vi "Teleop.vi"(10 "Match Info":T2={"Autonomous Elapsed Seconds"=0.0, "TeleOp Elapsed Seconds"=0.0, "Disabled Elapsed Seconds"=0.0, "Visited Autonomous"=FALSE, "Visited TeleOp"=FALSE, "Visited Disabled"=FALSE, "Autonomous Settings"={"Autonomous Style"=enum."Independent", "VI Refnum"=refnum}}, 11 "Call Context":T3) -> ()   [LabVIEW 2011]
doc: "This VI is called for each TeleOp packet received from the DS where the robot is not disabled. It is often used to read from the joysticks and update I/O or to update setpoints for timed control loops. It should complete and return within 20 milliseconds or it may miss DS packets."
uses:
  <vilib>/Rock Robotics/WPI/DriverStation/WPI_DriverStationDerivedRobotMode.ctl
  <vilib>/Rock Robotics/WPI/DriverStation/WPI_DriverStationMatch Info.ctl
  <vilib>/Rock Robotics/WPI/Joystick/WPI_JoystickButtonState.ctl
  Robot Global Data.vi
panel:
  in  "rpm fender diff":dbl=900.0
  out "Buttons 2":T1
  in  "dedband":dbl=0.1 step=0.01
  out "drive 2":bool
  out "drive 1":bool
  out "x-y":u32
  in  "Numeric":dbl=0.3
  out "Buttons":T1
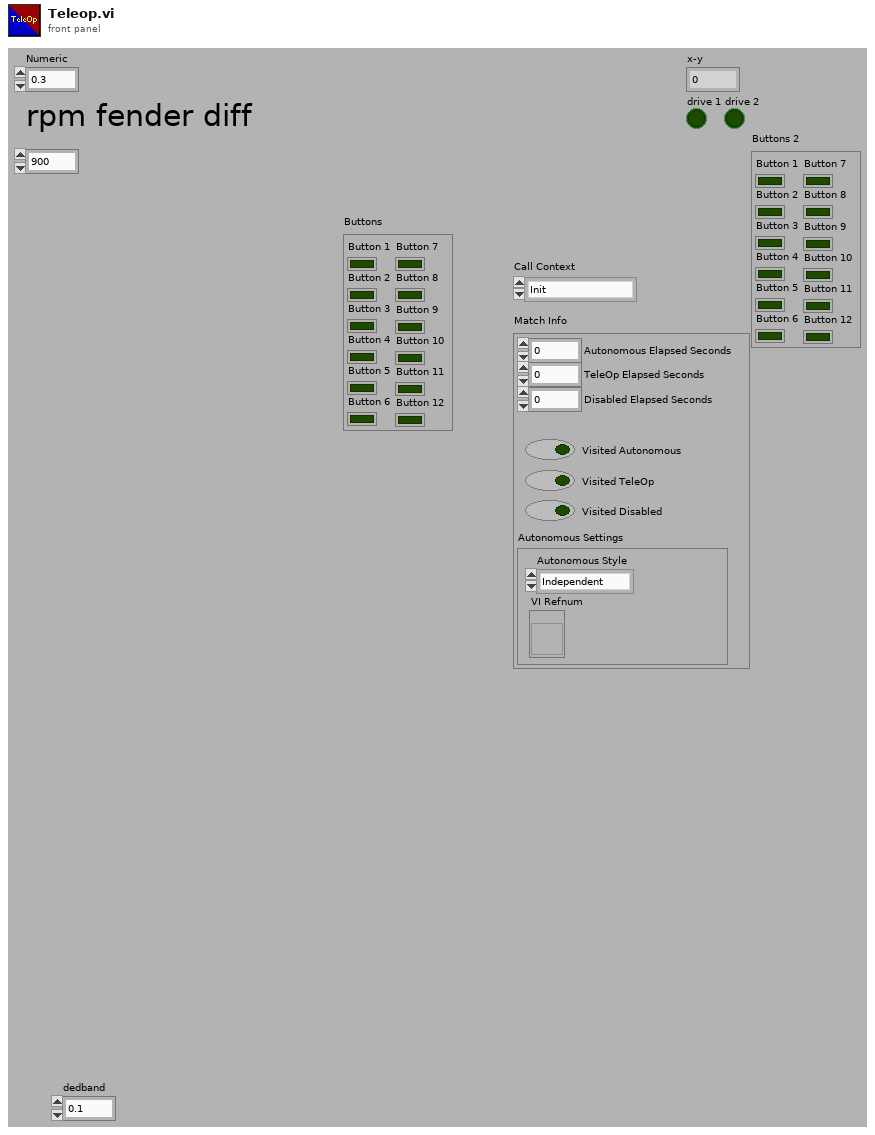
[diagram p1: front panel]
types:
  T1 = typedef "WPI_JoystickButtonState.ctl" = cluster{"Button 1":bool, "Button 2":bool, "Button 3":bool, "Button 4":bool, "Button 5":bool, "Button 6":bool, "Button 7":bool, "Button 8":bool, "Button 9":bool, "Button 10":bool, "Button 11":bool, "Button 12":bool}
  T2 = typedef "WPI_DriverStationMatch Info.ctl" = cluster{"Autonomous Elapsed Seconds":dbl, "TeleOp Elapsed Seconds":dbl, "Disabled Elapsed Seconds":dbl, "Visited Autonomous":bool, "Visited TeleOp":bool, "Visited Disabled":bool, "Autonomous Settings":cluster{"Autonomous Style":enum16{"Iterative", "Independent"}, "VI Refnum":refnum<vi>}}
  T3 = typedef "WPI_DriverStationDerivedRobotMode.ctl" = enum16{"Init", "Execute", "Stop"}
  T4 = typedef "WPI_JoystickDevRef.ctl" = cluster{"Device":T5}
  T5 = typedef "WPI_JoystickDeviceEnum.ctl" = enum16{"USB 1", "USB 2", "USB 3", "USB 4", "Kinect 1", "Kinect 2"}
  T6 = cluster{"axis 1 (x)":dbl, "axis 2 (y)":dbl, "axis 3 (throttle)":dbl, "axis 4":dbl, "axis 5":dbl, "axis 6":dbl}
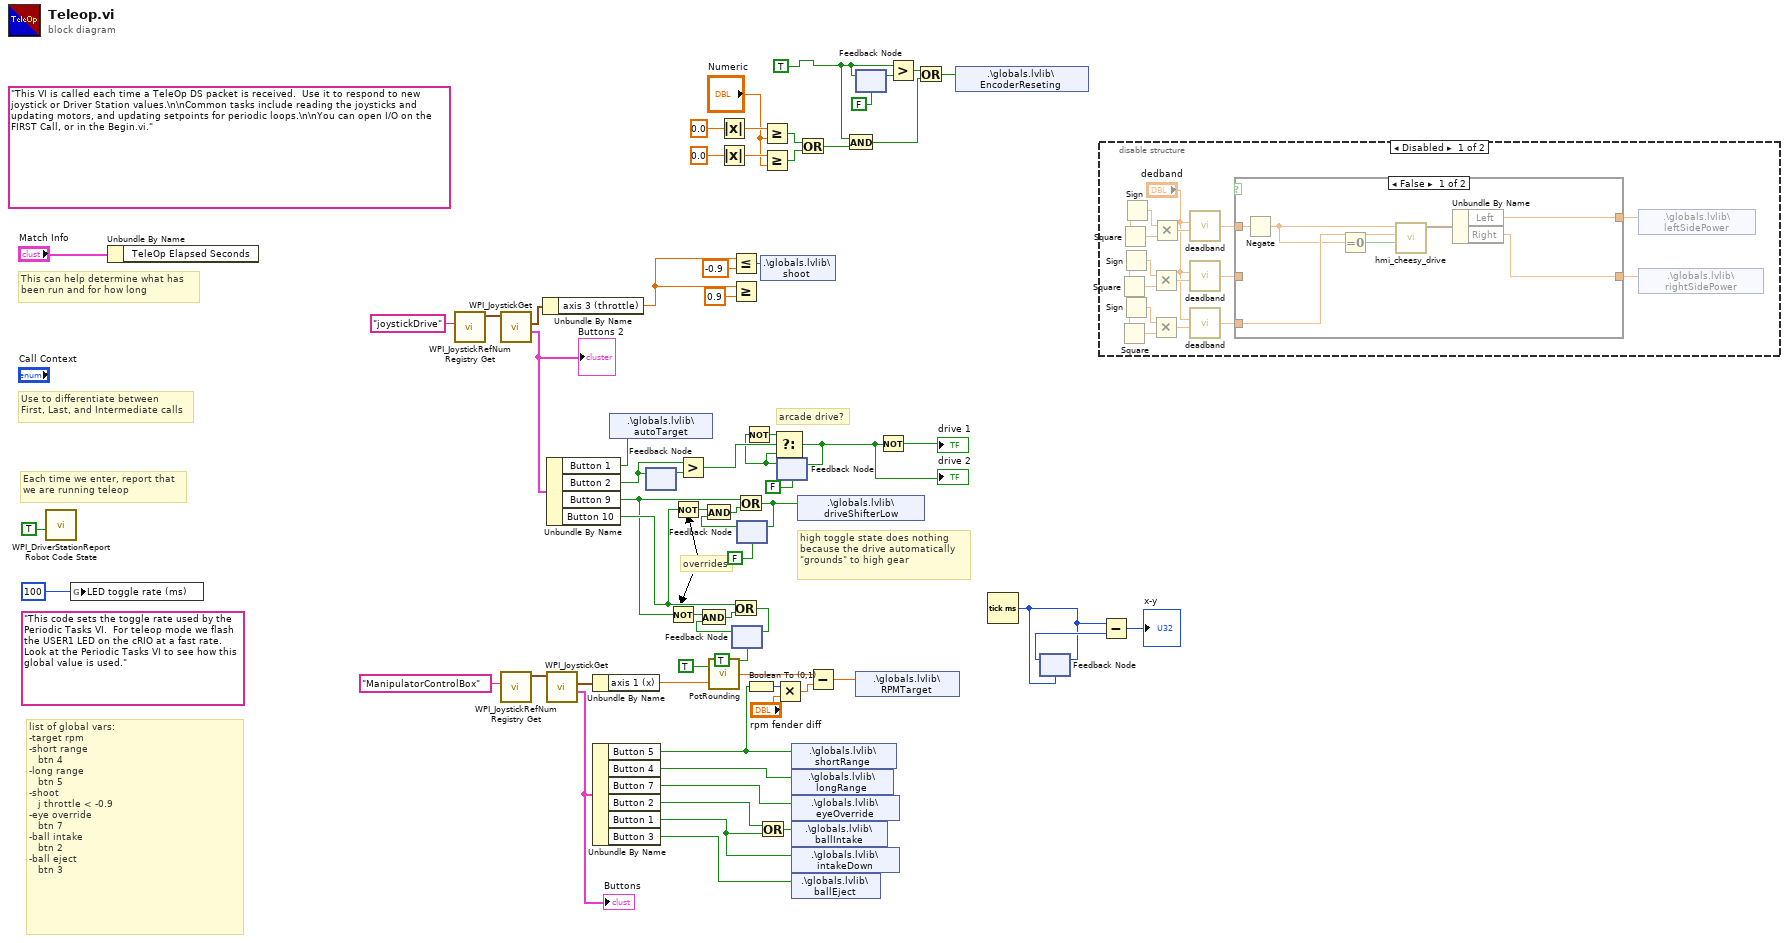
[diagram p0: block diagram]
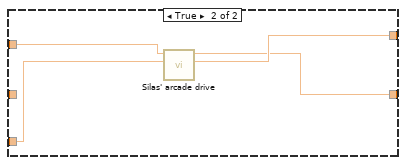
[diagram p2: hidden frame]
diagram:
  w20 = TRUE ("x")
  (unwired) "This code sets the toggle rate used by the Periodic Tasks VI.  For teleop mode we flash the USER1 LED on the cRIO at a fast rate.  Look at the Periodic Tasks VI to see how this global value is used."
  (unwired) "This VI is called each time a TeleOp DS packet is received.  Use it to respond to new joystick or Driver Station values.\n\nCommon tasks include reading the joysticks and updating motors, and updating setpoints for periodic loops.\n\nYou can open I/O on the FIRST Call, or in the Begin.vi."
  # "arcade drive?"
  # "high toggle state does nothing because the drive automatically \"grounds\" to high gear"
  # "overrides"
  # "list of global vars:\n-target rpm\n-short range\n   btn 4\n-long range\n   btn 5\n-shoot\n   j throttle < -0.9\n-eye override\n   btn 7\n-ball intake\n   btn 2\n-ball eject\n   btn 3"
  # "Each time we enter, report that\nwe are running teleop"
  # "Use to differentiate between\nFirst, Last, and Intermediate calls"
  # "This can help determine what has\nbeen run and for how long"
  n1 = call <vilib>:"WPI_DriverStationReport Robot Code State.vi"("TeleOp"=TRUE ("Autonomous")) -> ()  [unwired: 10 in, 1 out]
  n2 = global write "Robot Global Data.vi" "LED toggle rate (ms)"(u32 100 ("LED ms toggle rate")) -> ()
  n3 = Unbundle By Name("Match Info") -> ()  [unwired: 1 out]
  n4 = call <vilib>:"WPI_JoystickRefNum Registry Get.vi"("refnum name"="joystickDrive") -> ("JoystickDevRef"=w62:T4)  [unwired: 9 in, 1 out]
  n5 = call <vilib>:"WPI_JoystickGet.vi"("JoystickDevRef"=w62) -> ("Buttons"=w49:T1, "Axes"=w60:T6)  [unwired: 4 in, 1 out]
  "Buttons 2" <- w49
  n6 = call <vilib>:"WPI_JoystickRefNum Registry Get.vi"("refnum name"="ManipulatorControlBox") -> ("JoystickDevRef"=w61:T4)  [unwired: 9 in, 1 out]
  n7 = Unbundle By Name(w60) -> ("axis 3 (throttle)"=w17:dbl)
  n8 = Unbundle By Name(w49) -> ("Button 1"=w28:bool, "Button 2"=w26:bool, "Button 9"=w25:bool, "Button 10"=w52:bool)
  n9 = call <vilib>:"WPI_JoystickGet.vi"("JoystickDevRef"=w61) -> ("Buttons"=w58:T1, "Axes"=w59:T6)  [unwired: 4 in, 1 out]
  "Buttons" <- w58
  n10 = Unbundle By Name(w59) -> ("axis 1 (x)"=w46:dbl)
  n11 = Unbundle By Name(w58) -> ("Button 5"=w6:bool, "Button 4"=w57:bool, "Button 7"=w7:bool, "Button 2"=w14:bool, "Button 1"=w13:bool, "Button 3"=w12:bool)
  n12 = shared-variable ".\\globals.lvlib\\autoTarget"(w28) -> ()  [unwired: 1 in, 1 out]
  n13 = feedback-in #1(w26) -> ()
  n14 = feedback #1() -> (w27:bool)  [unwired: 1 in]
  n15 = Not(x=w25) -> (.not. x?=w55:bool)
  n16 = Not(x=w52) -> (.not. x?=w54:bool)
  n17 = Greater?(x=w26, y=w27) -> (0:w24:bool)
  n18 = call "PotRounding.vi"("Potentiometer"=w46, "Invert?"=TRUE) -> ("shooter output"=w2:dbl)
  n19 = Absolute Value(x=0.0) -> (abs(x)=w40:dbl)
  n20 = Absolute Value(x=0.0) -> (abs(x)=w39:dbl)
  n21 = Less Or Equal?(x=w17, y=-0.9) -> (x <= y?=w19:bool)
  n22 = Greater Or Equal?(x=w17, y=0.9) -> ()  [unwired: 1 out]
  n23 = feedback #2(TRUE) -> (w48:bool)
  n24 = And(x=w55, y=w48) -> (x .and. y?=w56:bool)
  n25 = Or(x=w52, y=w56) -> (x .or. y?=w44:bool)
  n26 = feedback-in #2(w44) -> ()
  n27 = feedback #3(FALSE) -> (w50:bool)
  n28 = And(x=w54, y=w50) -> (x .and. y?=w53:bool)
  n29 = Or(x=w25, y=w53) -> (x .or. y?=w43:bool)
  n30 = feedback-in #3(w43) -> ()
  n31 = Boolean To (0,1)(Boolean=w6) -> (0, 1=w5:i16)
  n32 = Or(x=w14, y=w13) -> (x .or. y?=w15:bool)
  n33 = shared-variable ".\\globals.lvlib\\shoot"(w19) -> ()  [unwired: 1 in, 1 out]
  n34 = Greater Or Equal?(x=w40, y="Numeric") -> (x >= y?=w37:bool)
  n35 = Greater Or Equal?(x=w39, y="Numeric") -> (x >= y?=w36:bool)
  n36 = Multiply(x=w5, y="rpm fender diff") -> (x*y=w1:dbl)
  n37 = feedback #4(FALSE) -> (w21:bool)
  n38 = Not(x=w21) -> (.not. x?=w22:bool)
  n39 = Select(t=w22, s=w24, f=w21) -> (s? t:f=w10:bool)
  "drive 2" <- w10
  n40 = feedback-in #4(w10) -> ()
  n41 = shared-variable ".\\globals.lvlib\\shortRange"(w6) -> ()  [unwired: 1 in, 1 out]
  n42 = shared-variable ".\\globals.lvlib\\longRange"(w57) -> ()  [unwired: 1 in, 1 out]
  n43 = shared-variable ".\\globals.lvlib\\eyeOverride"(w7) -> ()  [unwired: 1 in, 1 out]
  n44 = shared-variable ".\\globals.lvlib\\ballIntake"(w15) -> ()  [unwired: 1 in, 1 out]
  n45 = shared-variable ".\\globals.lvlib\\intakeDown"(w13) -> ()  [unwired: 1 in, 1 out]
  n46 = shared-variable ".\\globals.lvlib\\ballEject"(w12) -> ()  [unwired: 1 in, 1 out]
  n47 = Or(x=w37, y=w36) -> (x .or. y?=w35:bool)
  n48 = shared-variable ".\\globals.lvlib\\driveShifterLow"(w43) -> ()  [unwired: 1 in, 1 out]
  n49 = Subtract(x=w2, y=w1) -> (x-y=w3:dbl)
  n50 = And(x=w20, y=w35) -> (x .and. y?=w41:bool)
  n51 = feedback #5(FALSE) -> (w34:bool)
  n52 = feedback-in #5(w20) -> ()
  n53 = shared-variable ".\\globals.lvlib\\RPMTarget"(w3) -> ()  [unwired: 1 in, 1 out]
  n54 = Not(x=w10) -> (.not. x?=→"drive 1":bool)
  n55 = Greater?(x=w20, y=w34) -> (0:w33:bool)
  n56 = Or(x=w33, y=w41) -> (x .or. y?=w32:bool)
  n57 = shared-variable ".\\globals.lvlib\\EncoderReseting"(w32) -> ()  [unwired: 1 in, 1 out]
  n58 = Tick Count (ms)() -> (millisecond timer value=w30:u32)
  n59 = feedback #6(w30) -> (w31:u32)
  n60 = feedback-in #6(w30) -> ()
  n61 = disable-structure shown="Disabled" {
    frame Disabled {
      n62 = Square() -> (x=w69:dbl, x^2=w71:dbl)
      n63 = Sign() -> (0:w84:dbl, 1:w78:dbl)
      n64 = Square(x=w78) -> (x^2=w85:dbl)
      n65 = Sign(1:w69) -> (0:w72:dbl)
      n66 = Sign() -> (0:w82:dbl, 1:w79:dbl)
      n67 = Square(x=w79) -> (x^2=w83:dbl)
      n68 = Multiply(x=w84, y=w85) -> (x*y=w81:dbl)
      n69 = Multiply(x=w72, y=w71) -> (x*y=w73:dbl)
      n70 = Multiply(x=w82, y=w83) -> (x*y=w80:dbl)
      n71 = call "deadband.vi"("tolerance"="dedband", "input"=w80) -> ("output"=w77:dbl)  [unwired: 5 in]
      n72 = call "deadband.vi"("tolerance"="dedband", "input"=w81) -> ("output"=w76:dbl)  [unwired: 5 in]
      n73 = call "deadband.vi"("tolerance"="dedband", "input"=w73) -> ("output"=w68:dbl)  [unwired: 5 in]
      n74 = case shown="False" {
        selector: _ -> [_ _]
        tunnel: w77 -> [w87 w96]
        tunnel: w76 -> [_ _]
        tunnel: [w90 w95] -> w75
        tunnel: [w89 w94] -> w74
        tunnel: w68 -> [w92 w93]
        frame False {
          n75 = Negate(x=w87) -> (-x=w86:dbl)
          n76 = Equal To 0?(x=w86) -> (x = 0?=w88:bool)
          n77 = call "hmi_cheesy_drive.vi"("Quick Turn"=w88, "Wheel"=w92, "Throttle"=w86) -> ("Drive Data"=w91:cluster{"Left":dbl, "Right":dbl})  [unwired: 8 in]
          n78 = Unbundle By Name(w91) -> ("Left"=w90:dbl, "Right"=w89:dbl)
        }
        frame True {
          n79 = call "Silas' arcade drive.vi"("Right"=w93, "Left"=w96) -> ("Right"=w95:dbl, "Left"=w94:dbl)  [unwired: 8 in]
        }
      }
      n80 = shared-variable ".\\globals.lvlib\\leftSidePower"(w75) -> ()  [unwired: 1 in, 1 out]
      n81 = shared-variable ".\\globals.lvlib\\rightSidePower"(w74) -> ()  [unwired: 1 in, 1 out]
    }
    frame Enabled {
    }
  }
  n82 = Subtract(x=w30, y=w31) -> (x-y=→"x-y":u32)
